vi "Magnet.vi"(10 "milliseconds to wait":u32, 11 "on_off":bool) -> ()   [LabVIEW 2020]
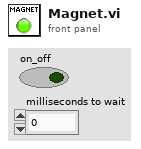
[diagram p1: front panel]
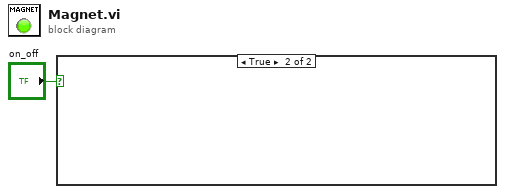
[diagram p0: block diagram]
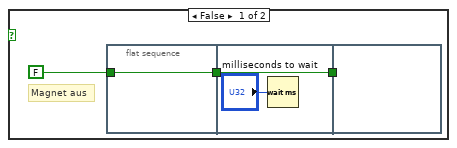
[diagram p2: hidden frame]
diagram:
  n1 = case shown="True" "on_off" {
    frame False {
      # "Magnet aus"
      n2 = flat-sequence {
        tunnel: FALSE ("DO0") -> [w5]
        tunnel: [w5] -> w3
        tunnel: w3 -> [w7]
        tunnel: [w7] -> w2
        tunnel: w2 -> [_]
        frame #0 {
        }
        frame #1 {
          n3 = Wait (ms)(milliseconds to wait="milliseconds to wait") -> ()  [unwired: 1 out]
        }
        frame #2 {
        }
      }
    }
    frame True {
    }
  }
